vi "Draw.vi"(0 "FSM.Annotation in":refnum<class "FSM.Annotation.lvclass">, 5 "picture in":picture, 7 "Label rect":T1, 11 "error in (no error)":errorcluster) -> (4 "FSM.Annotation out":refnum<class "FSM.Annotation.lvclass">, 6 "picture out":picture, 15 "error out":errorcluster)   [LabVIEW 2015, in "FSM.Annotation.lvclass"]
uses:
  FSM.Annotation.lvclass
  FSM.Annotation.lvclass/FSM.Annotation.ctl
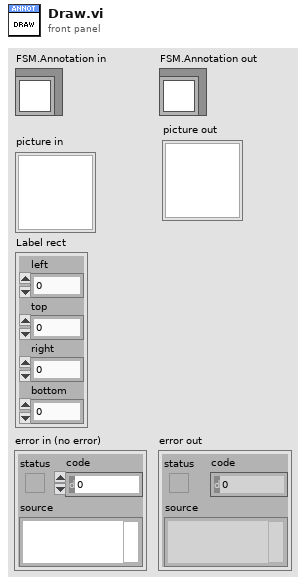
[diagram p1: front panel]
types:
  T1 = cluster{"left":i16, "top":i16, "right":i16, "bottom":i16}
  T2 = enum16{"User-specified Font", "Application Font", "System Font", "Dialog Font"}
  T3 = cluster{"Font Name:":string, "Size":i16, "Strikeout?":bool, "Italic?":bool, "Underline?":bool, "Outline?":bool, "Shadow?":bool, "Bold?":bool}
  T4 = cluster{"horizontal":enum16{"left", "center", "right"}, "vertical":enum16{"top", "center", "bottom"}}
  T5 = cluster{"Name":string, "Style":enum16{"Plain", "On", "Off", "On-Off"}}[]
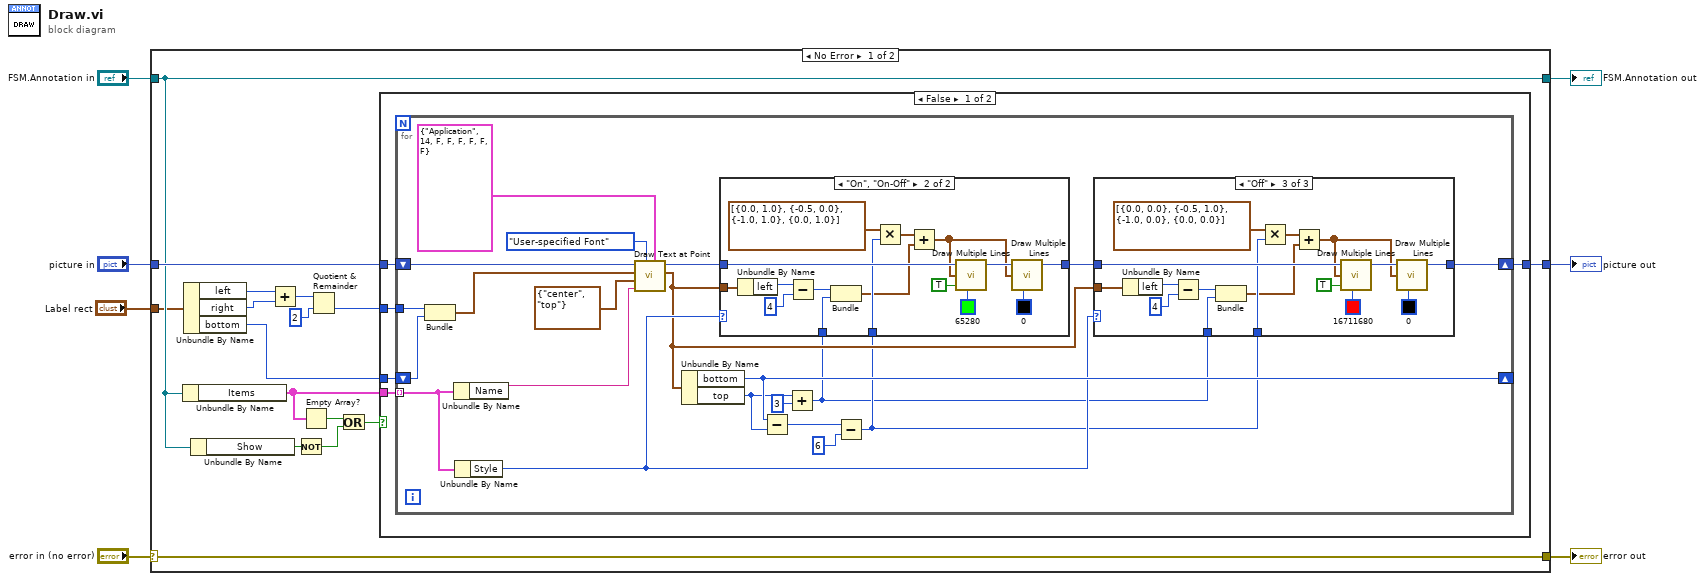
[diagram p0: block diagram]
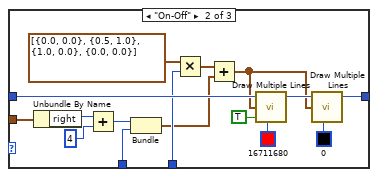
[diagram p3: hidden frame]
diagram:
  n1 = case shown="No Error" "error in (no error)" {
    selector: "error in (no error)" -> [w23 w103]
    tunnel: [w23 w103] -> w6
    tunnel: [w17 w102] -> w4
    tunnel: "FSM.Annotation in" -> [w17 w102]
    tunnel: "picture in" -> [w19 w101]
    tunnel: [w18 w101] -> w2
    tunnel: "Label rect" -> [w10 _]
    frame No Error {
      n2 = Unbundle By Name(w17) -> ("Items"=w20:T5)
      n3 = Unbundle By Name(w10) -> ("left"=w11:i16, "right"=w12:i16, "bottom"=w8:i16)
      n4 = Unbundle By Name(w17) -> ("Show"=w16:bool)
      n5 = Add(x=w11, y=w12) -> (x+y=w13:i16)
      n6 = Not(x=w16) -> (.not. x?=w15:bool)
      n7 = Empty Array?(array=w20) -> (empty?=w22:bool)
      n8 = Quotient & Remainder(x=w13, y=2) -> (floor(x/y)=w9:i32)  [unwired: 1 out]
      n9 = Or(x=w22, y=w15) -> (x .or. y?=w21:bool)
      n10 = case shown="False" w21 {
        tunnel: w20 -> [w28 _]
        tunnel: w19 -> [w27 w100]
        tunnel: [w26 w100] -> w18
        tunnel: w9 -> [w25 _]
        tunnel: w8 -> [w24 _]
        frame False {
          n11 = for {
            tunnel: w28 -> [w35] mode=indexing
            shift-right: [w36] -> w26
            shift-left: w27 -> [w49]
            tunnel: w25 -> [w44]
            shift-right: [w40] -> _
            shift-left: w24 -> [w43]
            n12 = Bundle(w44, "bottom"=w43) -> (w47:cluster{i32, "bottom":i16})  [unwired: 1 in]
            n13 = Unbundle By Name(w35) -> ("Name"=w42:string)
            n14 = Unbundle By Name(w35) -> ("Style"=w34:enum16{"Plain", "On", "Off", "On-Off"})
            n15 = call <vilib>:"Draw Text at Point.vi"("[user-specified font]"=T3 {"Font Name:"="Application", "Size"=14, "Strikeout?"=FALSE, "Italic?"=FALSE, "Underline?"=FALSE, "Outline?"=FALSE, "Shadow?"=FALSE, "Bold?"=FALSE}, "desired font(Application)"=T2."User-specified Font", "text"=w42, "alignment(left, top)"=T4 {"horizontal"=enum."center", "vertical"=enum."top"}, "origin"=w47, "picture"=w49) -> ("text rect"=w33:T1, "new picture"=w41:picture)  [unwired: 4 in]
            n16 = Unbundle By Name(w33) -> ("bottom"=w40:i16, "top"=w31:i16)
            n17 = Subtract(x=w40, y=w31) -> (x-y=w38:i16)
            n18 = Add(x=w31, y=i16 3) -> (x+y=w30:i16)
            n19 = Subtract(x=w38, y=i16 6) -> (x-y=w32:i16)
            n20 = case shown="\"On\", \"On-Off\"" w34 {
              tunnel: w41 -> [w83 w96]
              tunnel: w33 -> [_ w97]
              tunnel: [w83 w86] -> w37
              tunnel: w32 -> [_ w91]
              tunnel: w30 -> [_ w94]
              frame "Plain", Default {
              }
              frame "On", "On-Off" {
                n21 = Unbundle By Name(w97) -> ("left"=w98:i16)
                n22 = Subtract(x=w98, y=i16 4) -> (x-y=w99:i16)
                n23 = Bundle(w99, w94) -> (w89:cluster{i16, i16})  [unwired: 1 in]
                n24 = Multiply(x=cluster{dbl, dbl}[] [{0.0, 1.0}, {-0.5, 0.0}, {-1.0, 1.0}, {0.0, 1.0}], y=w91) -> (x*y=w90:cluster{dbl, dbl}[])
                n25 = Add(x=w90, y=w89) -> (x+y=w85:cluster{dbl, dbl}[])
                n26 = call <vilib>:"Draw Multiple Lines.vi"("picture"=w96, "line endpoints"=w85, "fill?(F)"=TRUE, "color(black)"=u32 65280) -> ("new picture"=w87:picture)  [unwired: 5 in]
                n27 = call <vilib>:"Draw Multiple Lines.vi"("picture"=w87, "line endpoints"=w85, "color(black)"=u32 0) -> ("new picture"=w86:picture)  [unwired: 6 in]
              }
            }
            n28 = case shown="\"Off\"" w34 {
              tunnel: w37 -> [w50 w63 w79]
              tunnel: w33 -> [_ w64 w80]
              tunnel: [w50 w53 w69] -> w36
              tunnel: w32 -> [_ w58 w74]
              tunnel: w30 -> [_ w61 w77]
              frame "Plain", Default {
              }
              frame "On-Off" {
                n29 = Unbundle By Name(w64) -> ("right"=w65:i16)
                n30 = Add(x=w65, y=i16 4) -> (x+y=w66:i16)
                n31 = Bundle(w66, w61) -> (w56:cluster{i16, i16})  [unwired: 1 in]
                n32 = Multiply(x=cluster{dbl, dbl}[] [{0.0, 0.0}, {0.5, 1.0}, {1.0, 0.0}, {0.0, 0.0}], y=w58) -> (x*y=w57:cluster{dbl, dbl}[])
                n33 = Add(x=w57, y=w56) -> (x+y=w52:cluster{dbl, dbl}[])
                n34 = call <vilib>:"Draw Multiple Lines.vi"("picture"=w63, "line endpoints"=w52, "fill?(F)"=TRUE, "color(black)"=u32 16711680) -> ("new picture"=w54:picture)  [unwired: 5 in]
                n35 = call <vilib>:"Draw Multiple Lines.vi"("picture"=w54, "line endpoints"=w52, "color(black)"=u32 0) -> ("new picture"=w53:picture)  [unwired: 6 in]
              }
              frame "Off" {
                n36 = Unbundle By Name(w80) -> ("left"=w81:i16)
                n37 = Subtract(x=w81, y=i16 4) -> (x-y=w82:i16)
                n38 = Bundle(w82, w77) -> (w72:cluster{i16, i16})  [unwired: 1 in]
                n39 = Multiply(x=cluster{dbl, dbl}[] [{0.0, 0.0}, {-0.5, 1.0}, {-1.0, 0.0}, {0.0, 0.0}], y=w74) -> (x*y=w73:cluster{dbl, dbl}[])
                n40 = Add(x=w73, y=w72) -> (x+y=w68:cluster{dbl, dbl}[])
                n41 = call <vilib>:"Draw Multiple Lines.vi"("picture"=w79, "line endpoints"=w68, "fill?(F)"=TRUE, "color(black)"=u32 16711680) -> ("new picture"=w70:picture)  [unwired: 5 in]
                n42 = call <vilib>:"Draw Multiple Lines.vi"("picture"=w70, "line endpoints"=w68, "color(black)"=u32 0) -> ("new picture"=w69:picture)  [unwired: 6 in]
              }
            }
          }
        }
        frame True {
        }
      }
    }
    frame Error {
    }
  }
  "error out" <- w6
  "FSM.Annotation out" <- w4
  "picture out" <- w2
